vi "Index Component Names.vi"(8 "Error In":errorcluster, 10 "Comp Name":string[](array[string]), 11 "Tab Page Ref":refnum<vi>[](array[refnum])) -> (0 "Error Out":errorcluster, 1 "Index Array":i32[][](array[numeric]), 3 "Tab Page Ref dup":refnum<vi>[](array[refnum]))   [LabVIEW 2014]
doc: "This VI find the name of components on each page of the Tab Cotnrol, and search the Componet Name array, stored in the TDMS file, to find the match. \n\nThe output is a 2D array in which each row collects the indeces of Component Name that corresponds with the page component name array."
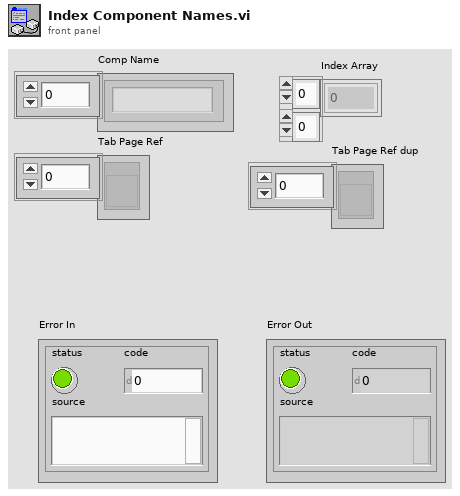
[diagram p1: front panel]
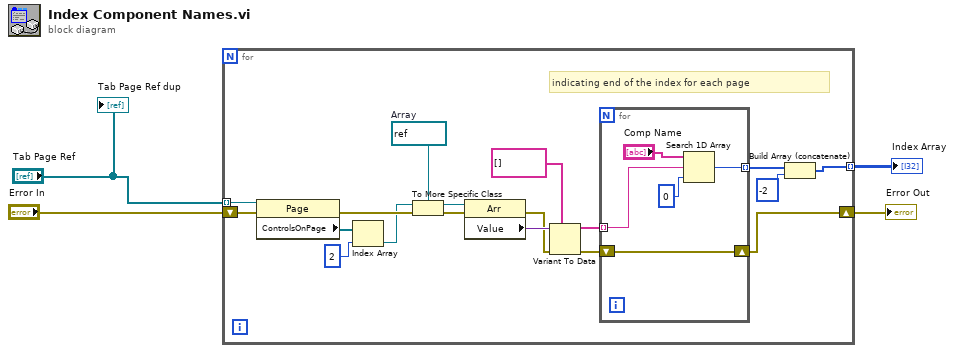
[diagram p0: block diagram]
diagram:
  n1 = for {
    tunnel: "Tab Page Ref" -> [w22] mode=indexing
    shift-right: [w8] -> w2
    shift-left: "Error In" -> [w21]
    tunnel: [w7] -> w1 mode=indexing
    w14 = refnum<vi> refnum  # Array
    # "indicating end of the index for each page"
    n2 = property class="Page"(reference=w22, error in=w21) -> (error out=w17:errorcluster, "ControlsOnPage"=w20:refnum<vi>[])  [unwired: 1 out]
    n3 = Index Array(array=w20, index=2) -> (element=w16:refnum<vi>)
    n4 = To More Specific Class(target class=w14, reference=w16, error in=w17) -> (specific class reference=w15:refnum<vi>, error out=w18:errorcluster)
    n5 = property class="Arr"(reference=w15, error in=w18) -> (error out=w11:errorcluster, "Value"=w13:variant)  [unwired: 1 out]
    n6 = Variant To Data(error in=w11, type=string[] [], Variant=w13) -> (data=w9:string[], error out=w10:errorcluster)
    n7 = for {
      shift-right: [w24] -> w8
      shift-left: w10 -> [w24]
      tunnel: w9 -> [w26] mode=indexing
      tunnel: [w23] -> w6 mode=indexing
      n8 = Search 1D Array(1D array="Comp Name", element=w26, start index (0)=0) -> (index of element=w23:i32)
    }
    n9 = Build Array (concatenate)(w6, -2 ("index")) -> (w7:i32[])
  }
  "Error Out" <- w2
  "Index Array" <- w1
  "Tab Page Ref dup" <- "Tab Page Ref"
